vi "CreatePrivateEvents.vi"(8 "error in (no error)":errorcluster, 11 "Plane":refnum<class "Plane.lvclass">) -> (0 "error out":errorcluster, 3 "Plane out":refnum<class "Plane.lvclass">)   [LabVIEW 2020, in "Plane.lvclass"]
doc: "---------------------------------------------------------------\nJKI State Machine Objects™\nhttp://jki.net/state-machine-objects/\nCopyright (C) 2005-2015, JKI <info@jki.net>\nALL RIGHTS RESERVEDJKI State Machine Objects (SMO) 1.0.0.4\nJKI - JKI\nCopyright (c) 2015, JKI"
uses:
  Plane.lvclass
  Plane.lvclass/Plane.ctl
  <vilib>/JKI/JKI SMO/SMO/SMO.lvclass
  Typedefs/PrivateEvents--Plane.SetLatitude.ctl
  Typedefs/PrivateEvents--Plane.SetLongitude.ctl
  Typedefs/PrivateEvents--Plane.SetCoord.ctl
  Typedefs/PrivateEvents--Plane.SetAltitude.ctl
  Typedefs/PrivateEvents--Plane.SetHeading.ctl
  Typedefs/PrivateEvents--Plane.SetSpeed.ctl
  Typedefs/PrivateEvents--Plane.SetICAO.ctl
  Typedefs/PrivateEvents--Plane.SetHDG.ctl
  Typedefs/PrivateEvents--Plane.GetPlaneData.ctl
  Typedefs/PrivateEvents--Plane.SetUpdateTime.ctl
panel:
  # "For instructions on how to use the JKI State Machine Objects, examples and video tutorials, visit:\nhttp://jki.net/state-machine-objects/\n\nJKI State Machine Objects™\nhttp://jki.net/state-machine-objects/\nCopyright (C) 2005-2015, JKI <info@jki.net>\nALL RIGHTS RESERVED"
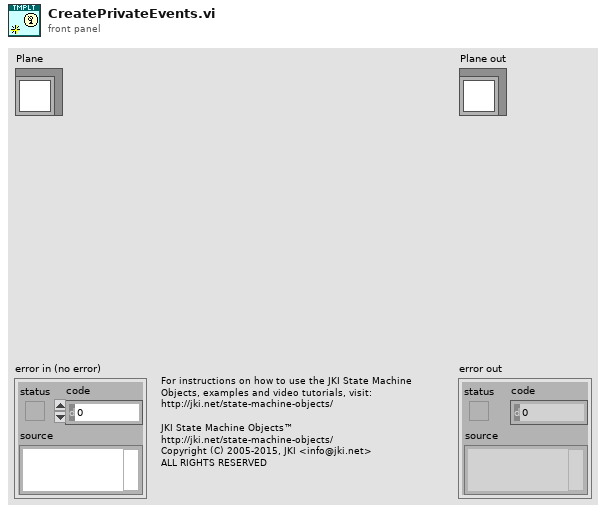
[diagram p1: front panel]
types:
  T1 = typedef "Plane.lvclass/PrivateData--Ref.ctl" = refnum<data-value>
  T2 = typedef "Plane.lvclass/PrivateEvents--Plane.SetUpdateTime.ctl" = timestamp
  T3 = typedef "Plane.lvclass/PrivateEvents--Plane.GetPlaneData.ctl" = cluster{"ICAO":string, "Lat":dbl, "Long":dbl, "Speed":dbl, "Heading":dbl, "Altitude":dbl, "LastUpdate":timestamp}
  T4 = typedef "Plane.lvclass/PrivateEvents--Plane.SetHDG.ctl" = dbl
  T5 = typedef "Plane.lvclass/PrivateEvents--Plane.SetICAO.ctl" = string
  T6 = typedef "Plane.lvclass/PrivateEvents--Plane.SetSpeed.ctl" = dbl
  T7 = typedef "Plane.lvclass/PrivateEvents--Plane.SetHeading.ctl" = bool
  T8 = typedef "Plane.lvclass/PrivateEvents--Plane.SetAltitude.ctl" = dbl
  T9 = typedef "Plane.lvclass/PrivateEvents--Plane.SetCoord.ctl" = cluster{"Lat":dbl, "Long":dbl}
  T10 = typedef "Plane.lvclass/PrivateEvents--Plane.SetLongitude.ctl" = bool
  T11 = typedef "Plane.lvclass/PrivateEvents--Plane.SetLatitude.ctl" = dbl
  T12 = typedef "Plane.lvclass/PrivateData--Cluster.ctl" = cluster{"Configuration":T13, "Public Events":T14, "Protected Events":T15, "Data":string, "Private Events":T16}
  T13 = typedef "Plane.lvclass/Configuration--Cluster.ctl" = cluster{"Suffix":string}
  T14 = typedef "Plane.lvclass/PublicEvents--Cluster.ctl" = cluster{"Data Changed":refnum<user-event>}
  T15 = typedef "Plane.lvclass/ProtectedEvents--Cluster.ctl" = cluster{"API_Template":refnum<user-event>}
  T16 = typedef "Plane.lvclass/PrivateEvents--Cluster.ctl" = cluster{"SetLatitude":refnum<user-event>, "SetLongitude":refnum<user-event>, "SetCoord":refnum<user-event>, "SetAltitude":refnum<user-event>, "SetHeading":refnum<user-event>, "SetSpeed":refnum<user-event>, "SetICAO":refnum<user-event>, "SetHDG":refnum<user-event>, "GetPlaneData":refnum<user-event>, "SetUpdateTime":refnum<user-event>}
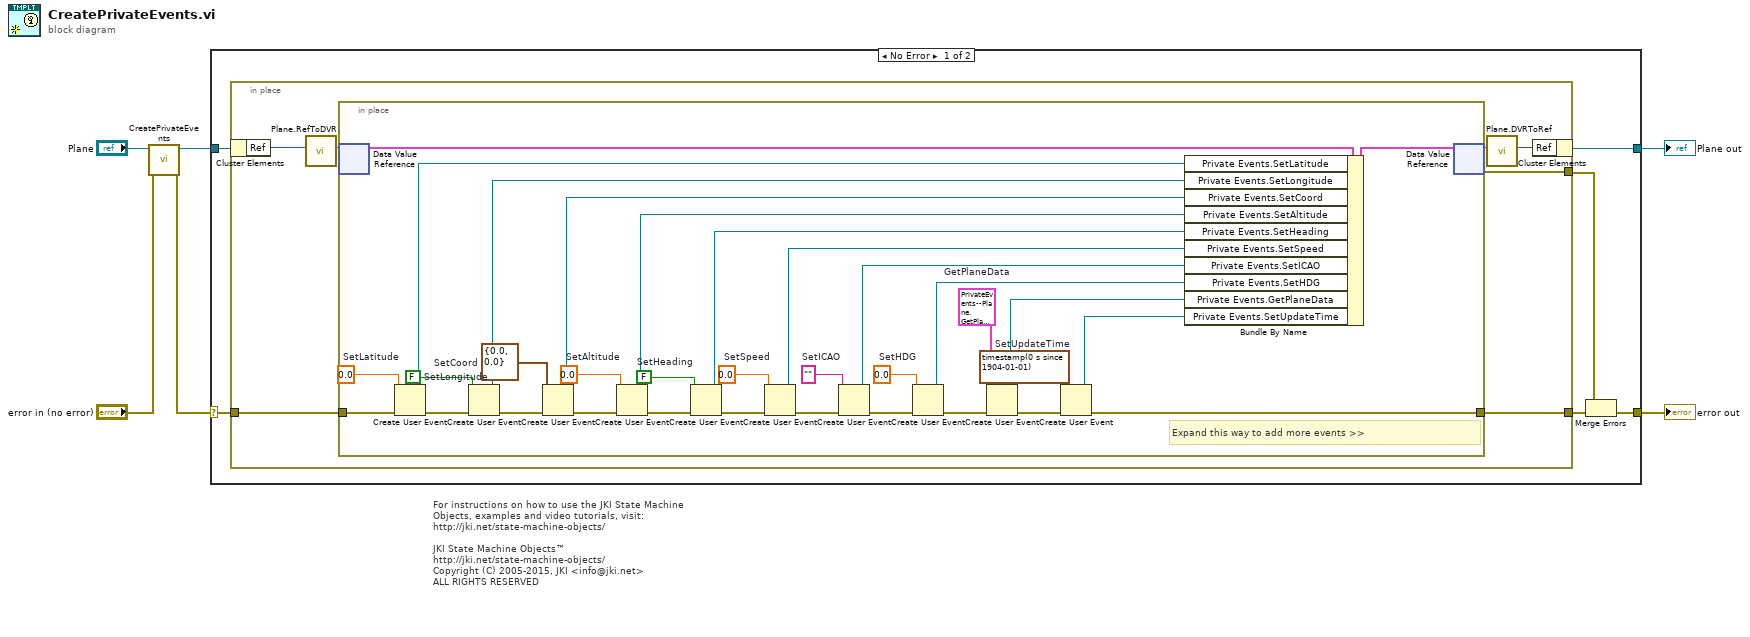
[diagram p0: block diagram]
diagram:
  # "For instructions on how to use the JKI State Machine Objects, examples and video tutorials, visit:\nhttp://jki.net/state-machine-objects/\n\nJKI State Machine Objects™\nhttp://jki.net/state-machine-objects/\nCopyright (C) 2005-2015, JKI <info@jki.net>\nALL RIGHTS RESERVED"
  n1 = call-parent "CreatePrivateEvents.vi"("error in (no error)"="error in (no error)", "SMO"="Plane") -> ("error out"=w1:errorcluster, "SMO out"=w3:refnum<class "Plane.lvclass">)  [unwired: 8 in]
  n2 = case shown="No Error" w1 {
    selector: w1 -> [w10 w54]
    tunnel: [w8 w54] -> w5
    tunnel: [w11 w53] -> w6
    tunnel: w3 -> [w12 w53]
    frame No Error {
      n3 = in-place {
        in-place-border: w10 -> [w19]
        in-place-border: [w16] -> w7
        in-place-border: [w15] -> w9
        n4 = in-place-cluster #1(w12) -> ("Ref"=w18:u32)
        n5 = call "Plane.RefToDVR.vi"("Ref"=w18) -> ("Ref"=w14:T1)  [unwired: 10 in]
        n6 = in-place {
          in-place-border: w19 -> [w52]
          in-place-border: [w22] -> w16
          w21 = T2 timestamp(0 s since 1904-01-01)  # SetUpdateTime
          w24 = T3 {"ICAO"="", "Lat"=0.0, "Long"=0.0, "Speed"=0.0, "Heading"=0.0, "Altitude"=0.0, "LastUpdate"=timestamp(0 s since 1904-01-01)}  # GetPlaneData
          w27 = T4 0.0  # SetHDG
          w30 = T5 ""  # SetICAO
          w33 = T6 0.0  # SetSpeed
          w36 = T7 FALSE  # SetHeading
          w39 = T8 0.0  # SetAltitude
          w42 = T9 {"Lat"=0.0, "Long"=0.0}  # SetCoord
          w45 = T10 FALSE  # SetLongitude
          w48 = T11 0.0  # SetLatitude
          # "Expand this way to add more events >>"
          n7 = in-place-dvr #2(w14) -> (w51:T12)  [unwired: 1 out]
          n8 = Create User Event(user event datatype=w48, error in=w52) -> (user event=w47:refnum<user-event>, error out=w49:errorcluster)
          n9 = Create User Event(user event datatype=w45, error in=w49) -> (user event=w44:refnum<user-event>, error out=w46:errorcluster)
          n10 = Create User Event(user event datatype=w42, error in=w46) -> (user event=w41:refnum<user-event>, error out=w43:errorcluster)
          n11 = Create User Event(user event datatype=w39, error in=w43) -> (user event=w38:refnum<user-event>, error out=w40:errorcluster)
          n12 = Create User Event(user event datatype=w36, error in=w40) -> (user event=w35:refnum<user-event>, error out=w37:errorcluster)
          n13 = Create User Event(user event datatype=w33, error in=w37) -> (user event=w32:refnum<user-event>, error out=w34:errorcluster)
          n14 = Create User Event(user event datatype=w30, error in=w34) -> (user event=w29:refnum<user-event>, error out=w31:errorcluster)
          n15 = Create User Event(user event datatype=w27, error in=w31) -> (user event=w26:refnum<user-event>, error out=w28:errorcluster)
          n16 = Create User Event(user event datatype=w24, error in=w28) -> (user event=w23:refnum<user-event>, error out=w25:errorcluster)
          n17 = Create User Event(user event datatype=w21, error in=w25) -> (user event=w20:refnum<user-event>, error out=w22:errorcluster)
          n18 = Bundle By Name(cluster=w51, "Private Events.SetLatitude"=w47, "Private Events.SetLongitude"=w44, "Private Events.SetCoord"=w41, "Private Events.SetAltitude"=w38, "Private Events.SetHeading"=w35, "Private Events.SetSpeed"=w32, "Private Events.SetICAO"=w29, "Private Events.SetHDG"=w26, "Private Events.GetPlaneData"=w23, "Private Events.SetUpdateTime"=w20) -> (w50:T12)
          n19 = in-place-dvr #2(w50) -> (w17:T1, w15:errorcluster)
        }
        n20 = call "Plane.DVRToRef.vi"("Ref"=w17) -> ("Ref"=w13:u32)  [unwired: 10 in]
        n21 = in-place-cluster #1("Ref"=w13) -> (w11:refnum<class "Plane.lvclass">)
      }
      n22 = Merge Errors(w9, w7) -> (w8:errorcluster)
    }
    frame Error {
    }
  }
  "error out" <- w5
  "Plane out" <- w6
